vi "Initialize AI.vi"(8 "error in":errorcluster, 11 "Channel":string="ai0") -> (0 "error out":errorcluster, 3 "task out":refnum<k21>)   [LabVIEW 2023, in "AI.lvlib"]
uses:
  AI.lvlib
  <vilib>/DAQmx/create/channels.llb/DAQmx Create Channel (AI-Voltage-Basic).vi
panel:
  in  "Task":string="A_Station2_DUT1"
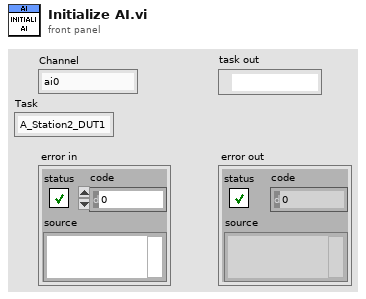
[diagram p1: front panel]
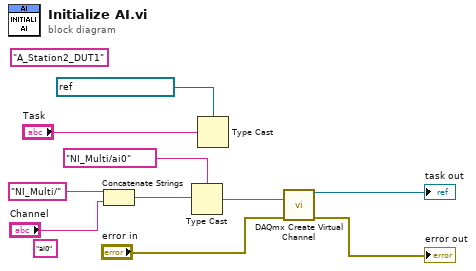
[diagram p0: block diagram]
diagram:
  (unwired) "A_Station2_DUT1" ("x")
  (unwired) "ai0" ("string")
  n1 = Concatenate Strings("NI_Multi/", "Channel") -> (w2:string)
  n2 = Type Cast(type=tag "NI_Multi/ai0" ("physical channels 3"), x=w2) -> (*(type *) &x=w1:tag)
  n3 = Type Cast(type=refnum<k21> "A_Station2_DUT1" ("task in"), x="Task") -> ()  [unwired: 1 out]
  n4 = call-poly <vilib>:"DAQmx Create Virtual Channel.vi"("physical channels"=w1, "error in"="error in") -> ("task out"=→"task out":refnum<k21>, "error out"=→"error out":errorcluster)  [unwired: 12 in]
